vi "BenchmarkNonReentrantAFE.vi"() -> ()   [LabVIEW 2017]
uses:
  AFE/Inputs.ctl
  AFE/Gains.ctl
  AFE/Range.ctl
  AFE/Setpoint.ctl
  AFE/Signals.ctl
  AFE/Parameters.ctl
  AFE/ManualControl.ctl
  AFE/Outputs.ctl
  <vilib>/NI/NonreentrantSinglePoint/Multiplier/Multiplier.lvclass
  <vilib>/NI/NonreentrantSinglePoint/Adder/Adder.lvclass
  <vilib>/NI/NonreentrantSinglePoint/Subtractor/Subtractor.lvclass
  <vilib>/NI/NonreentrantSinglePoint/SinCos/SinCos.lvclass
  <vilib>/NI/NonreentrantSinglePoint/Multiplier/Multiply0/Multiplier0.lvclass
  C:/Program Files (x86)/National Instruments/LabVIEW 2017/vi.lib/NI/NonreentrantSinglePoint/Multiplier/Multiplier.lvclass
  <vilib>/NI/NonreentrantSinglePoint/Divider/Divider0/Divider0.lvclass
  C:/Program Files (x86)/National Instruments/LabVIEW 2017/vi.lib/NI/NonreentrantSinglePoint/Divider/Divider.lvclass
  <vilib>/NI/NonreentrantSinglePoint/Adder/Adder0/Adder0.lvclass
  C:/Program Files (x86)/National Instruments/LabVIEW 2017/vi.lib/NI/NonreentrantSinglePoint/Adder/Adder.lvclass
  <vilib>/NI/NonreentrantSinglePoint/Subtractor/Subtractor0/Subtractor0.lvclass
  C:/Program Files (x86)/National Instruments/LabVIEW 2017/vi.lib/NI/NonreentrantSinglePoint/Subtractor/Subtractor.lvclass
  <vilib>/NI/NonreentrantSinglePoint/Divider/Divider.lvclass
  <vilib>/NI/NonreentrantSinglePoint/SinCos/SinCos0/SinCos0.lvclass
  C:/Program Files (x86)/National Instruments/LabVIEW 2017/vi.lib/NI/NonreentrantSinglePoint/SinCos/SinCos.lvclass
  <vilib>/rvi/Emulation/niFpgaGetClockAttributes.vi
  <vilib>/rvi/Emulation/niFpgaSctlEmulationGetInTimedLoop.vi
  <vilib>/rvi/Emulation/niFpgaEmulationReportErrorSimple.vi
  <vilib>/rvi/Emulation/niFpgaCriticalErrorInLSC.vi
  AFE/ActiveFrontEnd.lvlib
  <vilib>/NI/PowerElectronicsControl/SVPWM/SVPWM/SVPWM.lvlib
panel:
  out "SVPWM_Timing":cluster{"ON":u32, "OFF":u32}[](array[cluster])
  out "SVPWM_Sector":u8
  out "rate":u32
  out "Outputs":T1
  in  "ManualControl":T2
  in  "Parameters":T3
  in  "Signals":T4
  in  "Setpoints":T5
  in  "Range":T6={"PLL_PIRad_high"=inf, "PLL_PiRad_low"=inf, "IQcmd_high"=inf, "IQcmd_low"=inf, "IDcmd_high"=inf, "IDcmd_low"=inf, "VDcmd_high"=inf, "VDcmd_low"=inf, "VQmcd_high"=inf, "VQcmd_low"=inf}
  in  "Gains":T7
  in  "Inputs":T8
  # "Device Utilization\n---------------------------\nTotal Slices: 50.8% (6751 out of 13300)\nSlice Registers: 19.0% (20183 out of 106400)\nSlice LUTs: 36.5% (19440 out of 53200)\nBlock RAMs: 3.6% (5 out of 140)\nDSP48s: 0.5% (1 out of 220)"
  # "Latency 837"
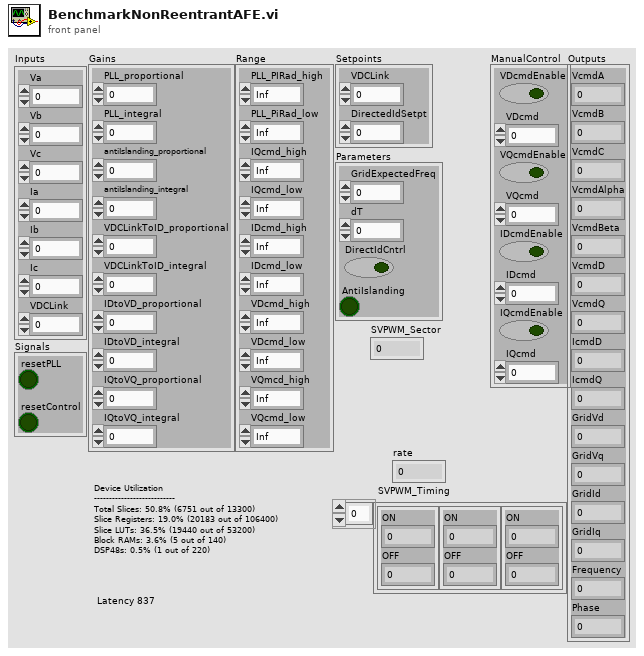
[diagram p1: front panel]
types:
  T1 = typedef "ActiveFrontEnd.lvlib/Outputs.ctl" = cluster{"VcmdA":sgl, "VcmdB":sgl, "VcmdC":sgl, "VcmdAlpha":sgl, "VcmdBeta":sgl, "VcmdD":sgl, "VcmdQ":sgl, "IcmdD":sgl, "IcmdQ":sgl, "GridVd":sgl, "GridVq":sgl, "GridId":sgl, "GridIq":sgl, "Frequency":sgl, "Phase":sgl}
  T2 = typedef "ActiveFrontEnd.lvlib/ManualControl.ctl" = cluster{"VDcmdEnable":bool, "VDcmd":sgl, "VQcmdEnable":bool, "VQcmd":sgl, "IDcmdEnable":bool, "IDcmd":sgl, "IQcmdEnable":bool, "IQcmd":sgl}
  T3 = typedef "ActiveFrontEnd.lvlib/Parameters.ctl" = cluster{"GridExpectedFreq":sgl, "dT":sgl, "DirectIdCntrl":bool, "AntiIslanding":bool}
  T4 = typedef "ActiveFrontEnd.lvlib/Signals.ctl" = cluster{"resetPLL":bool, "resetControl":bool}
  T5 = typedef "ActiveFrontEnd.lvlib/Setpoint.ctl" = cluster{"VDCLink":sgl, "DirectedIdSetpt":sgl}
  T6 = typedef "ActiveFrontEnd.lvlib/Range.ctl" = cluster{"PLL_PIRad_high":sgl, "PLL_PiRad_low":sgl, "IQcmd_high":sgl, "IQcmd_low":sgl, "IDcmd_high":sgl, "IDcmd_low":sgl, "VDcmd_high":sgl, "VDcmd_low":sgl, "VQmcd_high":sgl, "VQcmd_low":sgl}
  T7 = typedef "ActiveFrontEnd.lvlib/Gains.ctl" = cluster{"PLL_proportional":sgl, "PLL_integral":sgl, "antiIslanding_proportional":sgl, "antiIslanding_integral":sgl, "VDCLinkToID_proportional":sgl, "VDCLinkToID_integral":sgl, "IDtoVD_proportional":sgl, "IDtoVD_integral":sgl, "IQtoVQ_proportional":sgl, "IQtoVQ_integral":sgl}
  T8 = typedef "ActiveFrontEnd.lvlib/Inputs.ctl" = cluster{"Va":sgl, "Vb":sgl, "Vc":sgl, "Ia":sgl, "Ib":sgl, "Ic":sgl, "VDCLink":sgl}
  T9 = cluster{"Multiplier":refnum<class "Multiplier.lvclass">, "Divider":refnum<class "Divider.lvclass">, "Adder":refnum<class "Adder.lvclass">}
  T10 = cluster{"Multiplier":refnum<class "Multiplier.lvclass">, "Adder":refnum<class "Adder.lvclass">, "Subtractor":refnum<class "Subtractor.lvclass">, "SinCos":refnum<class "SinCos.lvclass">}
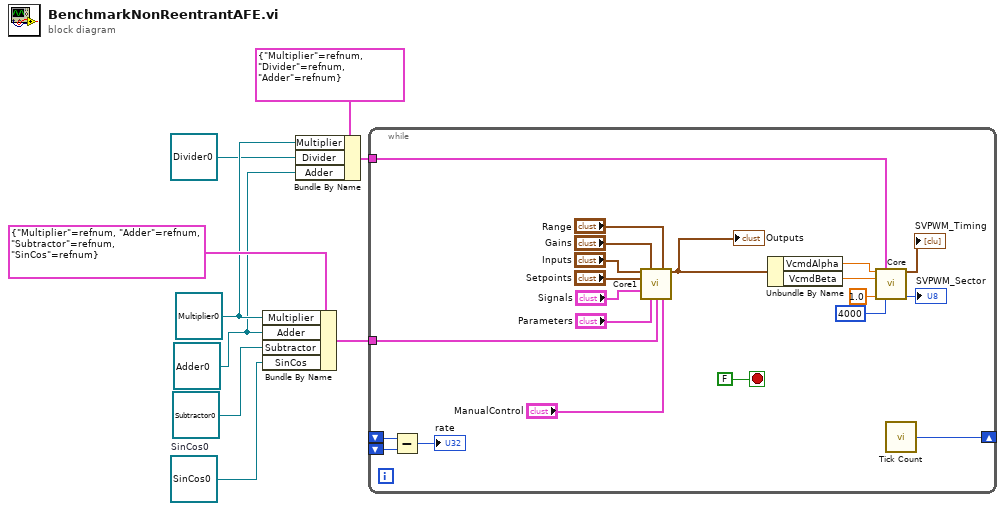
[diagram p0: block diagram]
diagram:
  w1 = refnum<class "SinCos0.lvclass"> refnum  # SinCos0
  w3 = refnum<class "Adder0.lvclass"> refnum ("Adder0.lvclass")
  w4 = refnum<class "Multiplier0.lvclass"> refnum ("Multiplier0.lvclass")
  n1 = Bundle By Name(cluster=T10 {"Multiplier"=refnum, "Adder"=refnum, "Subtractor"=refnum, "SinCos"=refnum} ("Resources"), "Multiplier"=w4, "Adder"=w3, "Subtractor"=refnum<class "Subtractor0.lvclass"> refnum ("Subtractor0.lvclass"), "SinCos"=w1) -> (w8:T10)
  n2 = Bundle By Name(cluster=T9 {"Multiplier"=refnum, "Divider"=refnum, "Adder"=refnum} ("Resource"), "Multiplier"=w4, "Divider"=refnum<class "Divider0.lvclass"> refnum ("Divider0.lvclass"), "Adder"=w3) -> (w6:T9)
  n3 = while {
    shift-right: [w22] -> _
    shift-left: _ -> [w20]
    shift-left: _ -> [w21]
    tunnel: w8 -> [w15]
    tunnel: w6 -> [w14]
    stop <- FALSE stop-if-true
    n4 = Subtract(x=w20, y=w21) -> (x-y=→"rate":u32)
    n5 = call "Core1.vi"("Inputs"="Inputs", "Gains"="Gains", "Range"="Range", "Setpoints"="Setpoints", "Signals"="Signals", "Parameters"="Parameters", "Resources"=w15, "ManualControl"="ManualControl") -> ("Outputs"=w18:T1)  [unwired: 7 in]
    "Outputs" <- w18
    n6 = Unbundle By Name(w18) -> ("VcmdAlpha"=w17:sgl, "VcmdBeta"=w16:sgl)
    n7 = call <vilib>:"Core.vi"("ref_alpha"=w17, "Resource"=w14, "ref_beta"=w16, "ref_max"=sgl 1.0, "Period"=u32 4000) -> ("SVPWM_Timing"=→"SVPWM_Timing":cluster{"ON":u32, "OFF":u32}[], "SVPWM_Sector"=→"SVPWM_Sector":u8)  [unwired: 9 in]
    n8 = call "Tick Count"() -> ("Tick Count(Ticks)"=w22:u32)
  }
